vi "Galil_programDownloadFile.vi"() -> ()   [LabVIEW 2011]
panel:
  in  "Galil.IGalil":refnum<k7>
  out "Library Version:":string
  out "LS Command Respons:":string
  out "error out":errorcluster
  out "Connected To:":string
  in  "Connection String:":string
  # "This vi Shows how to use the programDownload function of the Galil Communications Library.  \n\nIf Connection String is left blank, the vi will open the connections dialog when run.  If a value is input into Connection String, the vi will attempt to connect to the controller at that address (ie COM1 19200).\n\nThis vi downloads the program found in fileA.dmc to the controller, then uploads the program to fileB.dmc.\nLast it sends an LS command to the controller and displays the response"
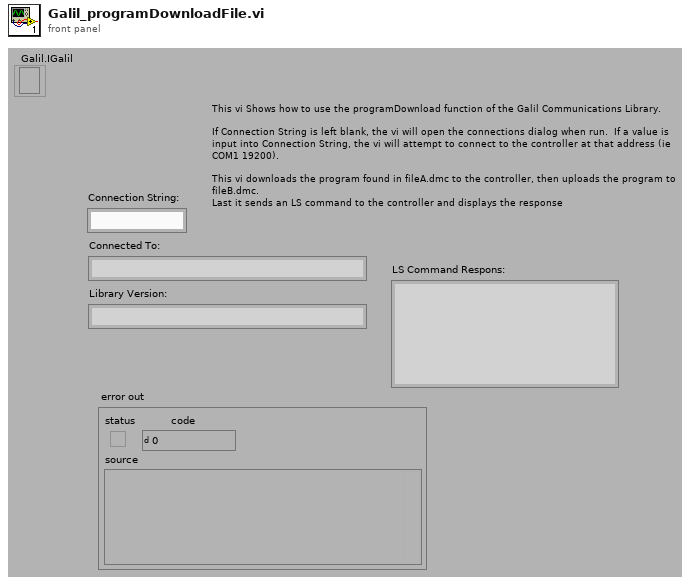
[diagram p1: front panel]
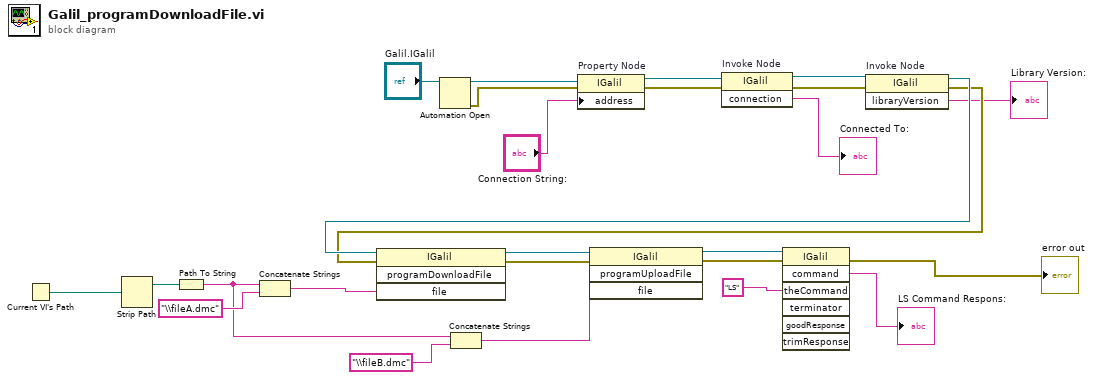
[diagram p0: block diagram]
diagram:
  n1 = Current VI's Path() -> (path=w8:path)
  n2 = Strip Path(path=w8) -> (stripped path=w7:path)  [unwired: 1 out]
  n3 = Path To String(path=w7) -> (string=w3:string)
  n4 = Concatenate Strings "Concatenate Strings"(w3, "\\fileA.dmc") -> (w5:string)
  n5 = Automation Open(Automation Refnum="Galil.IGalil") -> (Automation Refnum=w26:refnum<k7>, error out=w24:errorcluster)  [unwired: 1 in, 2 out]
  n6 = Concatenate Strings "Concatenate Strings"(w3, "\\fileB.dmc") -> (w4:string)
  n7 = property on="Property Node" class="IGalil"(reference=w26, error in=w24, "address"="Connection String:") -> (reference out=w25:refnum<k7>, error out=w23:errorcluster)
  n8 = invoke on="Invoke Node" class="IGalil" method="connection"(reference=w25, error in=w23) -> (reference out=w14:refnum<k7>, error out=w13:errorcluster, "connection"=→"Connected To:":string)  [unwired: 1 in]
  n9 = invoke on="Invoke Node" class="IGalil" method="libraryVersion"(reference=w14, error in=w13) -> (reference out=w12:refnum<k7>, error out=w11:errorcluster, "libraryVersion"=→"Library Version:":string)  [unwired: 1 in]
  n10 = invoke class="IGalil" method="programDownloadFile"(reference=w12, error in=w11, "file"=w5) -> (reference out=w20:refnum<k7>, error out=w19:errorcluster)  [unwired: 1 in, 2 out]
  n11 = invoke class="IGalil" method="programUploadFile"(reference=w20, error in=w19, "file"=w4) -> (reference out=w17:refnum<k7>, error out=w18:errorcluster)  [unwired: 1 in, 2 out]
  n12 = invoke class="IGalil" method="command"(reference=w17, error in=w18, "theCommand"="LS") -> (error out=→"error out":errorcluster, "command"=→"LS Command Respons:":string)  [unwired: 4 in, 5 out]
